vi "GetTxOn.vi"(6 "Legacy (f)?":bool, 8 "error in (no error)":errorcluster) -> (0 "error out":errorcluster, 2 "TxOn":bool[](array[boolean]), 5 "Timed Out?":bool)   [LabVIEW 2011]
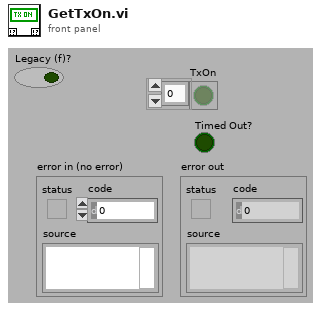
[diagram p1: front panel]
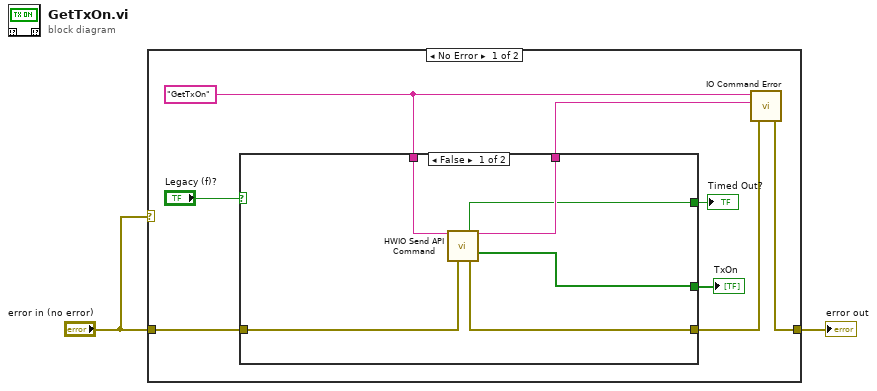
[diagram p0: block diagram]
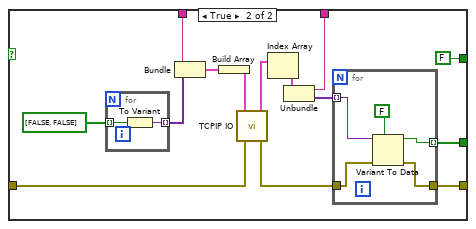
[diagram p2: hidden frame]
diagram:
  n1 = case shown="No Error" "error in (no error)" {
    tunnel: "error in (no error)" -> [w9 w38]
    tunnel: [w7 w38] -> w2
    frame No Error {
      w6 = "GetTxOn"
      n2 = case shown="False" "Legacy (f)?" {
        tunnel: [w14 w26] -> w10
        tunnel: w9 -> [w16 w25]
        tunnel: [w15 w23] -> w8
        tunnel: w6 -> [w12 w22]
        tunnel: [w13 w21] -> w5
        tunnel: [w11 FALSE ("Timed Out?")] -> w3
        frame False {
          n3 = call "HWIO Send API Command.vi"("Action"=w12, "error in (no error)"=w16) -> ("Timed Out?"=w11:bool, "Action out"=w13:string, "Boolean out"=w14:bool[], "error out"=w15:errorcluster)  [unwired: 6 in, 4 out]
        }
        frame True {
          n4 = for {
            tunnel: [w37] -> w29 mode=indexing
            tunnel: bool[] [FALSE, FALSE] -> [w36] mode=indexing
            n5 = To Variant(anything=w36) -> (Variant=w37:variant)
          }
          n6 = Bundle(w22, w29) -> (w30:cluster{string, variant[]})  [unwired: 1 out]
          n7 = Build Array(w30) -> (w18:cluster{string, variant[]}[])
          n8 = call "TCPIP IO.vi"("error in (no error)"=w25, "Commands"=w18) -> ("error out"=w24:errorcluster, "Responses"=w20:cluster{string, variant[]}[])  [unwired: 1 in, 3 out]
          n9 = Index Array(array=w20) -> (element=w19:cluster{string, variant[]})  [unwired: 1 in]
          n10 = Unbundle(w19) -> (w21:string, w27:variant[])
          n11 = for {
            tunnel: [w35] -> w23
            tunnel: w24 -> [w34]
            tunnel: w27 -> [w32] mode=indexing
            tunnel: [w31] -> w26 mode=indexing
            n12 = Variant To Data(error in=w34, type=FALSE, Variant=w32) -> (data=w31:bool, error out=w35:errorcluster)
          }
        }
      }
      "TxOn" <- w10
      "Timed Out?" <- w3
      n13 = call "IO Command Error.vi"("error in (no error)"=w8, "Command Returned (\"\")"=w5, "Command Sent (\"\")"=w6) -> ("error out"=w7:errorcluster)  [unwired: 4 out]
    }
    frame Error {
    }
  }
  "error out" <- w2
